vi "get_tracker_settings.vi"(1 "Cluster":T1) -> (0 "settings value cluster":T2)   [LabVIEW 2010]
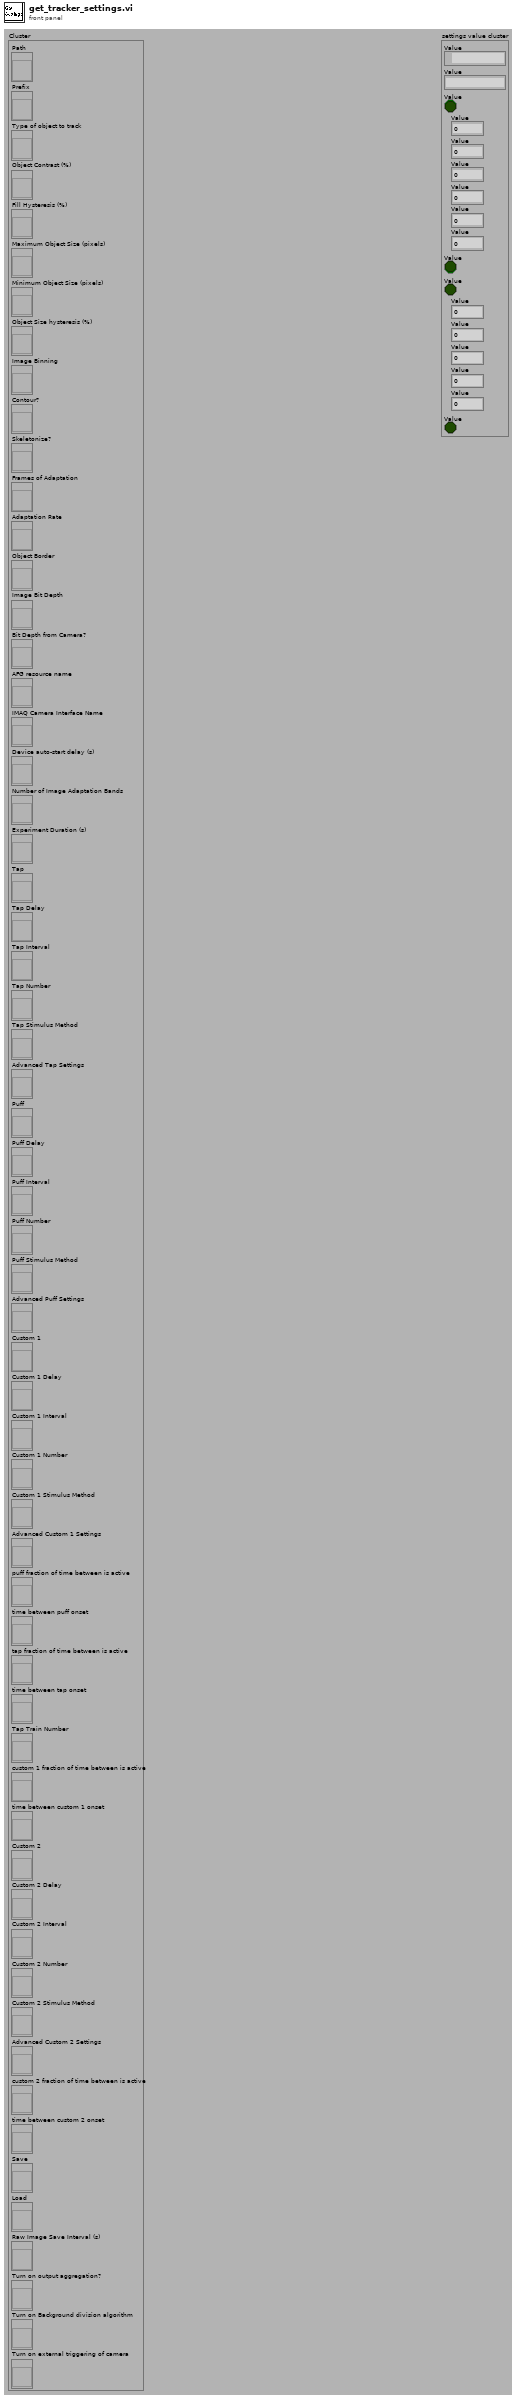
[diagram p1: front panel]
types:
  T1 = cluster{"Path":refnum<vi>, "Prefix":refnum<vi>, "Type of object to track":refnum<vi>, "Object Contrast (%)":refnum<vi>, "Fill Hysteresis (%)":refnum<vi>, "Maximum Object Size (pixels)":refnum<vi>, "Minimum Object Size (pixels)":refnum<vi>, "Object Size hysteresis (%)":refnum<vi>, "Image Binning":refnum<vi>, "Contour?":refnum<vi>, "Skeletonize?":refnum<vi>, "Frames of Adaptation":refnum<vi>, "Adaptation Rate":refnum<vi>, "Object Border":refnum<vi>, "Image Bit Depth":refnum<vi>, "Bit Depth from Camera?":refnum<vi>, "AFG resource name":refnum<vi>, "IMAQ Camera Interface Name":refnum<vi>, "Device auto-start delay (s)":refnum<vi>, "Number of Image Adaptation Bands":refnum<vi>, "Experiment Duration (s)":refnum<vi>, "Tap":refnum<vi>, "Tap Delay":refnum<vi>, "Tap Interval":refnum<vi>, "Tap Number":refnum<vi>, "Tap Stimulus Method":refnum<vi>, "Advanced Tap Settings":refnum<vi>, "Puff":refnum<vi>, "Puff Delay":refnum<vi>, "Puff Interval":refnum<vi>, "Puff Number":refnum<vi>, "Puff Stimulus Method":refnum<vi>, "Advanced Puff Settings":refnum<vi>, "Custom 1":refnum<vi>, "Custom 1 Delay":refnum<vi>, "Custom 1 Interval":refnum<vi>, "Custom 1 Number":refnum<vi>, "Custom 1 Stimulus Method":refnum<vi>, "Advanced Custom 1 Settings":refnum<vi>, "puff fraction of time between is active":refnum<vi>, "time between puff onset":refnum<vi>, "tap fraction of time between is active":refnum<vi>, "time between tap onset":refnum<vi>, "Tap Train Number":refnum<vi>, "custom 1 fraction of time between is active":refnum<vi>, "time between custom 1 onset":refnum<vi>, "Custom 2":refnum<vi>, "Custom 2 Delay":refnum<vi>, "Custom 2 Interval":refnum<vi>, "Custom 2 Number":refnum<vi>, "Custom 2 Stimulus Method":refnum<vi>, "Advanced Custom 2 Settings":refnum<vi>, "custom 2 fraction of time between is active":refnum<vi>, "time between custom 2 onset":refnum<vi>, "Save":refnum<vi>, "Load":refnum<vi>, "Raw Image Save Interval (s)":refnum<vi>, "Turn on output aggregation?":refnum<vi>, "Turn on Background division algorithm":refnum<vi>, "Turn on external triggering of camera":refnum<vi>}
  T2 = cluster{"Value":path, "Value":string, "Value":bool, "Value":dbl, "Value":dbl, "Value":i32, "Value":i32, "Value":dbl, "Value":u16, "Value":bool, "Value":bool, "Value":i32, "Value":i32, "Value":i32, "Value":u32, "Value":i32, "Value":bool}
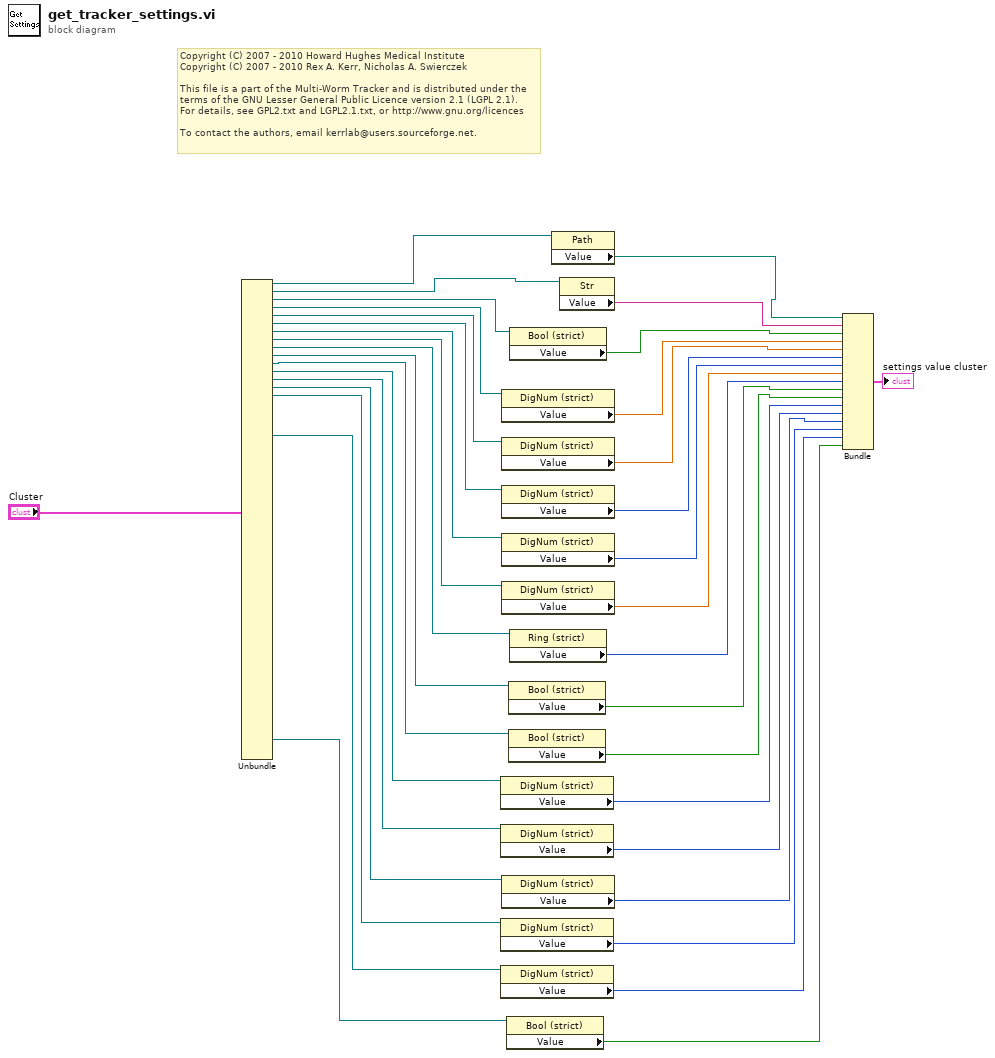
[diagram p0: block diagram]
diagram:
  # "Copyright (C) 2007 - 2010 Howard Hughes Medical Institute\nCopyright (C) 2007 - 2010 Rex A. Kerr, Nicholas A. Swierczek\n \nThis file is a part of the Multi-Worm Tracker and is distributed under the\nterms of the GNU Lesser General Public Licence version 2.1 (LGPL 2.1).\nFor details, see GPL2.txt and LGPL2.1.txt, or http://www.gnu.org/licences\n \nTo contact the authors, email kerrlab@users.sourceforge.net."
  n1 = Unbundle("Cluster") -> ("Path"=w36:refnum<vi>, "Prefix"=w35:refnum<vi>, "Type of object to track"=w26:refnum<vi>, "Object Contrast (%)"=w34:refnum<vi>, "Fill Hysteresis (%)"=w33:refnum<vi>, "Maximum Object Size (pixels)"=w32:refnum<vi>, "Minimum Object Size (pixels)"=w31:refnum<vi>, "Object Size hysteresis (%)"=w30:refnum<vi>, "Image Binning"=w29:refnum<vi>, "Contour?"=w18:refnum<vi>, "Skeletonize?"=w17:refnum<vi>, "Frames of Adaptation"=w14:refnum<vi>, "Adaptation Rate"=w10:refnum<vi>, "Object Border"=w9:refnum<vi>, "Image Bit Depth"=w8:refnum<vi>, "Number of Image Adaptation Bands"=w7:refnum<vi>, "Turn on output aggregation?"=w4:refnum<vi>)  [unwired: 43 out]
  n2 = property class="DigNum (strict)"(reference=w14) -> ("Value"=w13:i32)  [unwired: 1 in, 2 out]
  n3 = property class="DigNum (strict)"(reference=w10) -> ("Value"=w12:i32)  [unwired: 1 in, 2 out]
  n4 = property class="DigNum (strict)"(reference=w8) -> ("Value"=w6:u32)  [unwired: 1 in, 2 out]
  n5 = property class="DigNum (strict)"(reference=w7) -> ("Value"=w5:i32)  [unwired: 1 in, 2 out]
  n6 = property class="DigNum (strict)"(reference=w34) -> ("Value"=w24:dbl)  [unwired: 1 in, 2 out]
  n7 = property class="DigNum (strict)"(reference=w33) -> ("Value"=w23:dbl)  [unwired: 1 in, 2 out]
  n8 = property class="DigNum (strict)"(reference=w32) -> ("Value"=w22:i32)  [unwired: 1 in, 2 out]
  n9 = property class="DigNum (strict)"(reference=w31) -> ("Value"=w21:i32)  [unwired: 1 in, 2 out]
  n10 = property class="DigNum (strict)"(reference=w30) -> ("Value"=w20:dbl)  [unwired: 1 in, 2 out]
  n11 = property class="DigNum (strict)"(reference=w9) -> ("Value"=w11:i32)  [unwired: 1 in, 2 out]
  n12 = property class="Bool (strict)"(reference=w4) -> ("Value"=w3:bool)  [unwired: 1 in, 2 out]
  n13 = property class="Bool (strict)"(reference=w18) -> ("Value"=w16:bool)  [unwired: 1 in, 2 out]
  n14 = property class="Bool (strict)"(reference=w17) -> ("Value"=w15:bool)  [unwired: 1 in, 2 out]
  n15 = property class="Bool (strict)"(reference=w26) -> ("Value"=w25:bool)  [unwired: 1 in, 2 out]
  n16 = property class="Ring (strict)"(reference=w29) -> ("Value"=w19:u16)  [unwired: 1 in, 2 out]
  n17 = property class="Path"(reference=w36) -> ("Value"=w28:path)  [unwired: 1 in, 2 out]
  n18 = property class="Str"(reference=w35) -> ("Value"=w27:string)  [unwired: 1 in, 2 out]
  n19 = Bundle("Value"=w28, "Value"=w27, "Value"=w25, "Value"=w24, "Value"=w23, "Value"=w22, "Value"=w21, "Value"=w20, "Value"=w19, "Value"=w16, "Value"=w15, "Value"=w13, "Value"=w12, "Value"=w11, "Value"=w6, "Value"=w5, "Value"=w3) -> (→"settings value cluster":T2)  [unwired: 1 in]
